vi "pl1000OpenUnitAsync.vi"(8 "error in (no error)":errorcluster) -> (0 "error out":errorcluster, 3 "openStatus":T1(ring))   [LabVIEW 2016, in "pl1000.lvlib"]
uses:
  pl1000.lvlib
  pl1000.dll
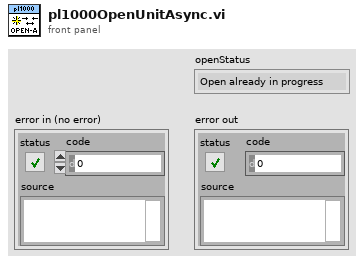
[diagram p1: front panel]
types:
  T1 = enum16{"Open already in progress", "Open initialized"}
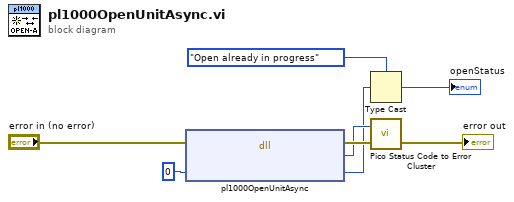
[diagram p0: block diagram]
diagram:
  n1 = dll-call lib="pl1000.dll" fn="pl1000OpenUnitAsync"(error in="error in (no error)", "openStatus"=i16 0 ("handle")) -> (error out=w7:errorcluster, "status"=w6:u32, "openStatus"=w2:i16)  [unwired: 2 in, 1 out]
  n2 = Type Cast(type=T1."Open already in progress", x=w2) -> (*(type *) &x=→"openStatus":T1)
  n3 = call "Pico Status Code to Error Cluster.vi"("error in"=w7, "PICO_STATUS"=w6) -> ("error out"=→"error out":errorcluster)  [unwired: 1 in]
